vi "Scan Engine Slot Page.vi"(8 "error in (no error)":errorcluster, 11 "Node Ptr":T3 format="%.0x") -> (0 "error out":errorcluster)   [LabVIEW 2019, in "SEECD System Explorer.lvlib"]
uses:
  SEECD System Explorer.lvlib
  <vilib>/NI VeriStand/Custom Device API/Custom Device Item Ref.ctl
  Includes/Modules.lvlibp/RSI Module/Module Models.ctl
  Includes/Modules.lvlibp/RSI Module/SubPanel Command.ctl
  Shared/Globals/Scan Engine GUIDs.vi
  <vilib>/NI VeriStand/Custom Device API/Custom Device API.lvlib
  Includes/Modules.lvlibp/RSI Module/RSI Module.lvclass
  Shared/SEECD Shared.lvlib
  Shared/Globals/Property Strings.vi
  Type Defs/Slot Programming Mode.ctl
panel:
  in  "Slot Programming Mode":T1
  out "Slot #":u32
  in  "Module":T2
  in  "Header":cluster{"Section Name":string}={"Section Name"="Slot Settings"}
  in  "Description":string
  out "Name":string
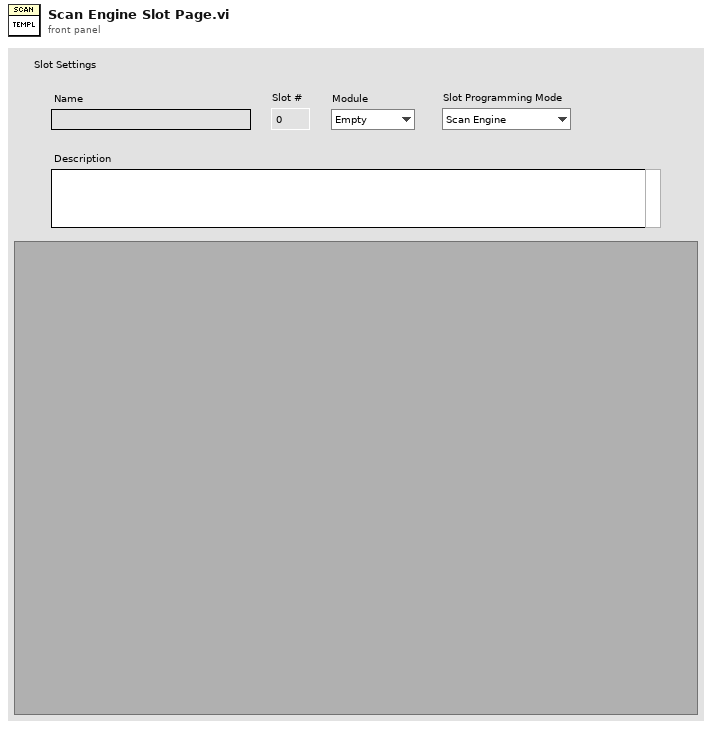
[diagram p1: front panel]
types:
  T1 = typedef "SEECD System Explorer.lvlib/Slot Programming Mode.ctl" = enum16{"Scan Engine", "LabVIEW FPGA", "NI-DAQmx", "Don't Modify"}
  T2 = typedef "Modules.lvlibp/RSI Module.lvclass/Module Models.ctl" = enum16{"Empty", "NI 9201", "NI 9203", "NI 9205", "NI 9206", "NI 9207", "NI 9208", "NI 9209", "NI 9210", "NI 9211", "NI 9212", "NI 9213", "NI 9214", "NI 9215", "NI 9216", "NI 9217", "NI 9219", "NI 9220", "NI 9221", "NI 9222", "NI 9223", "NI 9224", "NI 9225", "NI 9226", "NI 9227", "NI 9228", "NI 9229", "NI 9233", "NI 9234", "NI 9235", "NI 9236", "NI 9237", "NI 9239", "NI 9242", "NI 9244", "NI 9253", "NI 9263", "NI 9264", "NI 9265", "NI 9266", "NI 9269", "NI 9344", "NI 9350", "NI 9375", "NI 9401", "NI 9402", "NI 9403", "NI 9411", "NI 9421", "NI 9422", "NI 9423", "NI 9425", "NI 9426", "NI 9435", "NI 9436", "NI 9437", "NI 9472", "NI 9474", "NI 9475", "NI 9476", "NI 9477", "NI 9478", "NI 9481", "NI 9482", "NI 9485"}
  T3 = typedef "Custom Device API.lvlib/Custom Device Item Ref.ctl" = u64
  T4 = enum8{"Enabled", "Disabled", "Disabled and Grayed Out"}
  T5 = typedef "Custom Device API.lvlib/Custom Device Item Info.ctl" = cluster{"Name":string, "Is Channel":bool, "GUID":string, "Is Waveform":bool}
  T6 = typedef "Modules.lvlibp/RSI Module.lvclass/SubPanel Command.ctl" = enum16{"Stop"}
  T7 = typedef "Custom Device API.lvlib/Custom Device Commands.ctl" = enum16{"Default", "Item renamed", "Shutdown", "Dynamic button pressed"}
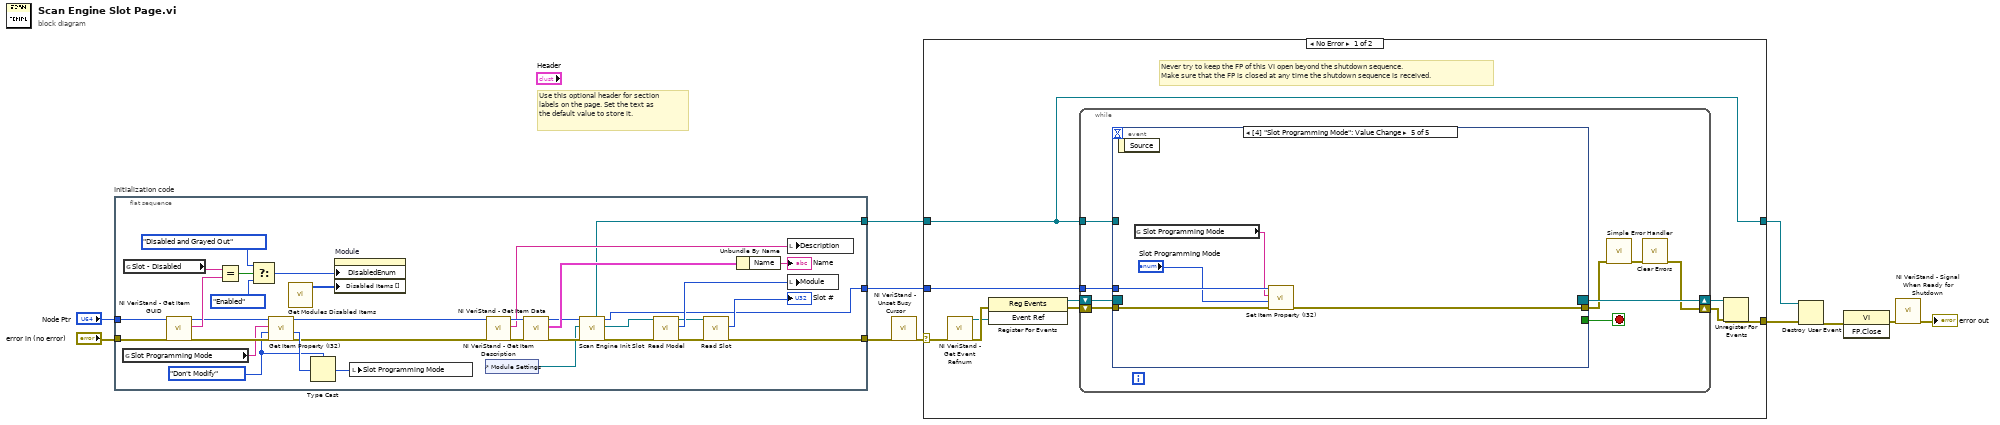
[diagram p0: block diagram]
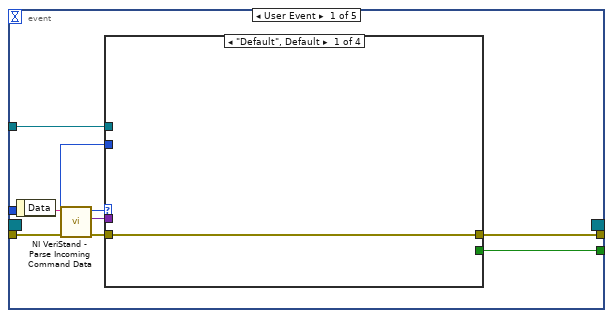
[diagram p2: hidden frame]
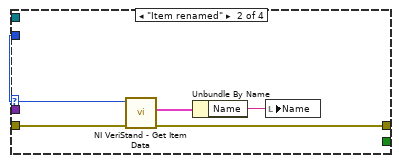
[diagram p3: hidden frame]
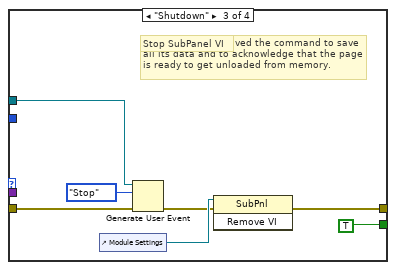
[diagram p4: hidden frame]
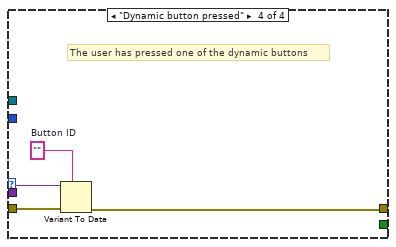
[diagram p5: hidden frame]
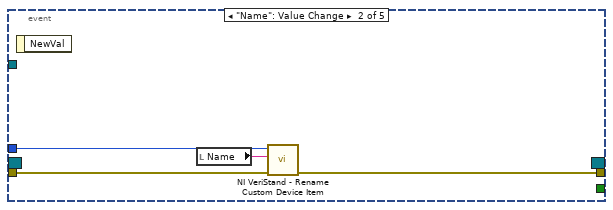
[diagram p6: hidden frame]
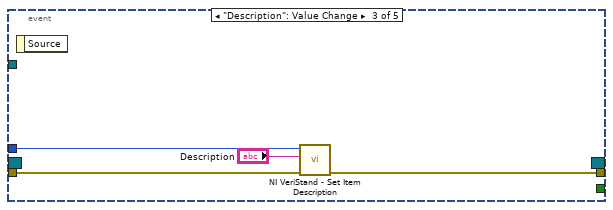
[diagram p7: hidden frame]
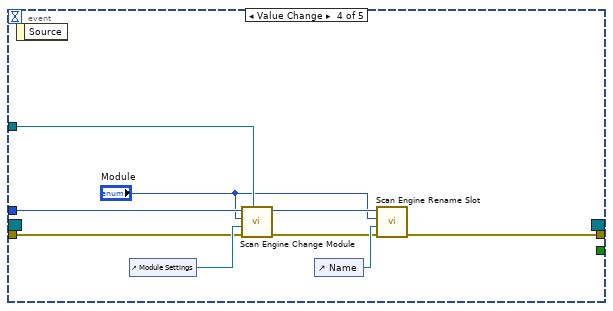
[diagram p8: hidden frame]
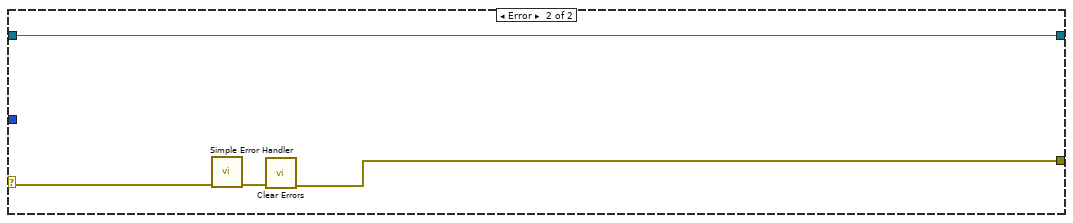
[diagram p9: hidden frame]
diagram:
  # "Use this optional header for section labels on the page. Set the text as the default value to store it."
  n1 = flat-sequence "Initialization code" {
    tunnel: "error in (no error)" -> [w27]
    tunnel: "Node Ptr" -> [w28]
    tunnel: [w29] -> w8
    tunnel: [w31] -> w6
    tunnel: [w33] -> w5
    frame #0 {
      w15 = Slot_Programming_Mode."Don't Modify" ("Slot Programming Mode 2")
      n2 = global read "Property Strings.vi" "Slot Programming Mode"() -> (w17:string)
      n3 = global read "Scan Engine GUIDs.vi" "Slot - Disabled"() -> (w26:string)
      n4 = call <vilib>:"NI VeriStand - Get Item GUID.vi"("error in (no error)"=w27, "Item Ref in"=w28) -> ("error out"=w19:errorcluster, "GUID"=w25:string, "Item Ref out"=w18:T3)  [unwired: 7 in]
      n5 = Equal?(x=w26, y=w25) -> (x = y?=w24:bool)
      n6 = Select(t=T4."Disabled and Grayed Out" ("Disabled"), s=w24, f=T4."Enabled" ("Disabled")) -> (s? t:f=w21:T4)
      n7 = call <vilib>:"Get Item Property (I32).vi"("error in (no error)"=w19, "Default Value"=w15, "Property Name"=w17, "Item Ref in"=w18) -> ("error out"=w13:errorcluster, "Value"=w16:i32, "Item Ref out"=w12:T3)  [unwired: 4 in, 1 out]
      n8 = call "Get Modules Disabled Items.vi"() -> ("DisabledItems[]"=w20:i32[])  [unwired: 11 in]
      n9 = Type Cast(type=w15, x=w16) -> (*(type *) &x=w14:T1)
      n10 = property on="Module" class="Enum (strict)"("DisabledEnum"=w21, "Disabled Items []"=w20) -> ()  [unwired: 2 in, 2 out]
      n11 = local write "Slot Programming Mode"(w14) -> ()
      n12 = control-ref of="Module Settings"() -> (w34:refnum<vi>)
      n13 = call <vilib>:"NI VeriStand - Get Item Description.vi"("error in (no error)"=w13, "Item Ref in"=w12) -> ("error out"=w43:errorcluster, "Description"=w44:string, "Item Ref out"=w45:T3)  [unwired: 7 out]
      n14 = call <vilib>:"NI VeriStand - Get Item Data.vi"("error in (no error)"=w43, "Item Ref in"=w45) -> ("error out"=w36:errorcluster, "Item Info"=w42:T5, "Item Ref out"=w35:T3)  [unwired: 7 out]
      n15 = call "Scan Engine Init Slot.vi"("error in (no error)"=w36, "SubPanel Ref"=w34, "Node Ptr In"=w35) -> ("error out"=w30:errorcluster, "RSI Module"=w32:refnum<class "RSI Module.lvclass">, "Node Ptr Out"=w31:T3, "SubPanel Command"=w33:refnum<user-event>)  [unwired: 5 in]
      n16 = call "Read Model.vi"("error in (no error)"=w30, "RSI Module in"=w32) -> ("error out"=w38:errorcluster, "Model"=w40:T2, "RSI Module out"=w39:refnum<class "RSI Module.lvclass">)  [unwired: 7 in]
      n17 = call "Read Slot.vi"("error in (no error)"=w38, "RSI Module in"=w39) -> ("error out"=w29:errorcluster, "Slot"=→"Slot #":u32)  [unwired: 7 in, 1 out]
      n18 = Unbundle By Name(w42) -> ("Name"=→"Name":string)
      n19 = local write "Description"(w44) -> ()
      n20 = local write "Module"(w40) -> ()
    }
  }
  n21 = call <vilib>:"NI VeriStand - Unset Busy Cursor.vi"("error in (no error)"=w8) -> ("error out"=w1:errorcluster)  [unwired: 10 out]
  n22 = case shown="No Error" w1 {
    selector: w1 -> [w47 w116]
    tunnel: [w52 w114] -> w3
    tunnel: w6 -> [w48 _]
    tunnel: w5 -> [w46 w113]
    tunnel: [w46 w113] -> w4
    frame No Error {
      # "Never try to keep the FP of this VI open beyond the shutdown sequence.\nMake sure that the FP is closed at any time the shutdown sequence is received."
      n23 = call <vilib>:"NI VeriStand - Get Event Refnum.vi"("error in (no error)"=w47) -> ("error out"=w55:errorcluster, "Event Ref"=w51:refnum<user-event>)  [unwired: 9 out]
      n24 = register-events(error in=w55, w51) -> (reference out=w49:refnum<event-registration>, error out=w50:errorcluster)  [unwired: 1 in]
      n25 = while {
        tunnel: w48 -> [w60]
        shift-right: [w57] -> w53
        shift-left: w50 -> [w63]
        shift-right: [w64] -> w54
        shift-left: w49 -> [w62]
        tunnel: w46 -> [w56]
        stop <- w61 stop-if-true
        n26 = event shown="[4] \"Slot Programming Mode\": Value Change" {
          selector: w62 -> [_ _ _ _ _]
          dyn-events: [_ _ _ _ _] -> w64
          timeout: _ -> [_ _ _ _ _]
          tunnel: w63 -> [w73 w94 w97 w104 w112]
          tunnel: [w69 _ _ _ _] -> w61
          tunnel: [w68 w93 w96 w99 w108] -> w59
          tunnel: w60 -> [w67 w92 w98 w103 w111]
          tunnel: w56 -> [w65 _ _ w105 _]
          event User Event {
            n27 = event-data() -> ("Data"=w72:string)  [unwired: 1 out]
            n28 = call <vilib>:"NI VeriStand - Parse Incoming Command Data.vi"("error in (no error)"=w73, "Incoming data"=w72) -> ("error out"=w71:errorcluster, "Outgoing data"=w66:variant, "Action"=w70:T7)  [unwired: 7 out]
            n29 = case shown="\"Default\", Default" w70 {
              tunnel: w71 -> [w74 w79 w83 w90]
              tunnel: [_ _ TRUE _] -> w69
              tunnel: [w74 w76 w80 w87] -> w68
              tunnel: w67 -> [_ w78 _ _]
              tunnel: w66 -> [_ _ _ w89]
              tunnel: w65 -> [_ _ w85 _]
              frame "Default", Default {
              }
              frame "Item renamed" {
                n30 = call <vilib>:"NI VeriStand - Get Item Data.vi"("error in (no error)"=w79, "Item Ref in"=w78) -> ("error out"=w76:errorcluster, "Item Info"=w77:T5)  [unwired: 8 out]
                n31 = Unbundle By Name(w77) -> ("Name"=w75:string)
                n32 = local write "Name"(w75) -> ()
              }
              frame "Shutdown" {
                # "Stop SubPanel VI"
                # "The page has received the command to save all its data and to acknowledge that the page is ready to get unloaded from memory."
                n33 = control-ref of="Module Settings"() -> (w82:refnum<vi>)
                n34 = Generate User Event(user event=w85, event data cluster=SubPanel_Command."Stop" ("event data"), error in=w83) -> (error out=w81:errorcluster)  [unwired: 1 in, 1 out]
                n35 = invoke class="SubPnl" method="Remove VI"(reference=w82, error in=w81) -> (error out=w80:errorcluster)  [unwired: 1 in, 2 out]
              }
              frame "Dynamic button pressed" {
                w88 = ""  # Button ID
                # "The user has pressed one of the dynamic buttons"
                n36 = Variant To Data(error in=w90, type=w88, Variant=w89) -> (error out=w87:errorcluster)  [unwired: 1 out]
              }
            }
          }
          event "Name": Value Change {
            n37 = event-data() -> ()  [unwired: 2 out]
            n38 = local read "Name"() -> (w91:string)
            n39 = call <vilib>:"NI VeriStand - Rename Custom Device Item.vi"("error in (no error)"=w94, "New Name"=w91, "Item Ref in"=w92) -> ("error out"=w93:errorcluster)  [unwired: 1 in, 7 out]
          }
          event "Description": Value Change {
            n40 = event-data() -> ()  [unwired: 2 out]
            n41 = call <vilib>:"NI VeriStand - Set Item Description.vi"("error in (no error)"=w97, "Description"="Description", "Item Ref in"=w98) -> ("error out"=w96:errorcluster)  [unwired: 8 out]
          }
          event Value Change {
            n42 = event-data() -> ()  [unwired: 2 out]
            n43 = control-ref of="Module Settings"() -> (w106:refnum<vi>)
            n44 = call "Scan Engine Change Module.vi"("SubPanel Event"=w105, "error in (no error)"=w104, "SubPanel Ref"=w106, "Module Model"="Module", "Node Ptr In"=w103) -> ("error out"=w100:errorcluster, "Node Ptr Out"=w102:T3)  [unwired: 5 in]
            n45 = control-ref of="Name"() -> (w107:refnum<vi>)
            n46 = call "Scan Engine Rename Slot.vi"("error in (no error)"=w100, "Name reference"=w107, "Module Model"="Module", "Node Ptr In"=w102) -> ("error out"=w99:errorcluster)  [unwired: 6 in, 1 out]
          }
          event Value Change {
            n47 = event-data() -> ()  [unwired: 2 out]
            n48 = global read "Property Strings.vi" "Slot Programming Mode"() -> (w109:string)
            n49 = call <vilib>:"Set Item Property (I32).vi"("error in (no error)"=w112, "Value"="Slot Programming Mode", "Property Name"=w109, "Item Ref in"=w111) -> ("error out"=w108:errorcluster)  [unwired: 5 in, 2 out]
          }
        }
        n50 = call <vilib>:"Simple Error Handler.vi"("error in (no error)"=w59) -> ("error out"=w58:errorcluster)  [unwired: 1 in, 7 out]
        n51 = call <vilib>:"Clear Errors.vi"("error in (no error)"=w58) -> ("error out"=w57:errorcluster)  [unwired: 1 in, 5 out]
      }
      n52 = Unregister For Events(event registration refnum=w54, error in=w53) -> (error out=w52:errorcluster)
    }
    frame Error {
      n53 = call <vilib>:"Simple Error Handler.vi"("error in (no error)"=w116) -> ("error out"=w115:errorcluster)  [unwired: 1 in, 7 out]
      n54 = call <vilib>:"Clear Errors.vi"("error in (no error)"=w115) -> ("error out"=w114:errorcluster)  [unwired: 1 in, 5 out]
    }
  }
  n55 = Destroy User Event(user event=w4, error in=w3) -> (error out=w2:errorcluster)
  n56 = invoke class="VI" method="FP.Close"(error in=w2) -> (error out=w11:errorcluster)  [unwired: 2 in, 2 out]
  n57 = call <vilib>:"NI VeriStand - Signal When Ready for Shutdown.vi"("error in (no error)"=w11) -> ("error out"=→"error out":errorcluster)  [unwired: 10 out]
